vi "Dissconnect.vi"(8 "error in (no error)":errorcluster, 11 "RemoteControl in":refnum<class "RemoteControl.lvclass">) -> (0 "error out":errorcluster, 3 "RemoteControl out":refnum<class "RemoteControl.lvclass">)   [LabVIEW 2019, in "RemoteControl.lvclass"]
uses:
  RemoteControl.lvclass
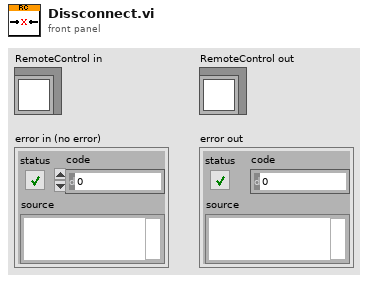
[diagram p1: front panel]
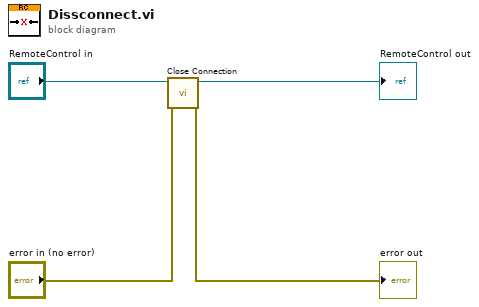
[diagram p0: block diagram]
diagram:
  n1 = call-dynamic "Close Connection.vi"("error in (no error)"="error in (no error)", "RemoteControl in"="RemoteControl in") -> ("error out"=→"error out":errorcluster, "RemoteControl out"=→"RemoteControl out":refnum<class "RemoteControl.lvclass">)  [unwired: 8 in]
